vi "20151004 Main_one action input .vi"() -> ()   [LabVIEW 2013]
uses:
  SSNN(super simple neural network)_2.1/Neural Network/Types/Stop Settings.ctl
  SSNN(super simple neural network)_2.1/Neural Network/Types/Error Evaluation.ctl
  <vilib>/MakerHub/LINX/Public/Sensors/Accelerometer/MPU60X0/DeviceAddresses.ctl
  controls/20151109 Action set.ctl
  controls/Pulse limit.ctl
  controls/Sample set.ctl
  SSNN(super simple neural network)_2.1/Neural Network/Types/Teaching Vector.ctl
  SSNN(super simple neural network)_2.1/Neural Network/Types/1D Array.ctl
  SSNN(super simple neural network)_2.1/Neural Network/Types/Neural Network.ctl
  SSNN(super simple neural network)_2.1/Neural Network/Types/2D Array.ctl
  SSNN(super simple neural network)_2.1/Neural Network/Types/Scaling Info.ctl
  SSNN(super simple neural network)_2.1/Neural Network/Super Simple Neural Network.lvlib
  <vilib>/MakerHub/LINX/Public/Sensors/Accelerometer/MPU60X0/MPU60X0.lvlib
panel:
  in  "Pulse limit":T1={"Pulse upper limit"=2400, "Pulse lower limit"=1500, "Fuzzy range"=50.0}
  out "Action chart":i16(graph)
  in  "Initial Pulse Widths (uS)":u16[](array[numeric])=[1100, 900, 2100, 1500, 1500, 600, 1600, 2100, 600, 1400, 700, 600] min=600 max=2400 step=100
  in  "Actions":T2=[-100, -50, -10, 0, 10, 50, 100]
  out "Pitch&Roll":T3(graph)={"Pitch"=1.64306105519083, "Roll"=-26.60639904187085, "Pulse"=1500.0, "Action"=0.0, "Pitch'"=0.0, "Roll'"=0.0, "Pulse'"=0.0}
  in  "Q learning setting":T4={"Pitch +limit"=15.0, "Pitch -limit"=-15.0, "Roll +limit"=5.0, "Roll -limit"=0.0, "Cost_c"=0.01, "Cost_0"=0.0, "Discounting factor"=1.0} {"Cost_0" format="%#_13g"; "Cost_c" format="%#_13g"}
  out "Cycles":i32=599
  in  "Neural network setting":T5={"Add Bias Inputs"=TRUE, "Output Layer Linear"=FALSE, "1st Hidden Layer"=10, "2nd Hidden Layer"=10, "# Inputs"=4, "Output Neurons/Outputs"=1}
  out "Error Trend":dbl[](graph)=[333.88049946998603, 84.67257917593295, 79.55145375361836, 165.88618567000654, 164.395409026523, 66.2860419585734, 89.94237535998712, 89.31153569817062, 48.467858482266436, 75.00403729966206, 75.0129349957244, 53.15644774430287, 49.173023491017965, 48.64104572122034, 47.03615785475572, 56.77040737122186, 56.73707087203033, 50.66515759517278, 46.94108756608759, 47.05005218060951, 49.10730725338338, 50.14010228928986, 49.105932754914605, 47.54849782076006, 46.130158362809, 45.14431666029949, 44.40933619615308, 43.21622556663465, 39.5637978090232, 41.311588761627874, 36.04355325175722, 32.85251820100693, 32.65212220800668, 28.980505575795966, 24.613605659371288, 22.04828944280029, 33.15201456870398, 19.751806387640762, 24.983784772589345, 20.123556544702225, 22.16816710032048, 24.761419168572694, 20.519403969578008, 22.075445422683597, 20.68097799083518, 21.774609704131727, 21.601837537514506, 21.08381595647031, 20.43182890729097, 22.04427690550854, 20.894295129000575, 20.106993070447466, 20.890368283068455, 21.208917859881538, 20.63770876867939, 21.091536913629373, 20.998527289682343, 20.795457971936926, 21.02597611803169, 20.227157731616355, 21.215734162324786, 20.650262532179397, 21.005392179444087, 20.725327488997934, 20.687878356478905, 20.855553191124425, 20.801611756610075, 20.738643649346614, 20.688105294347146, 20.838851997630606, 20.684708818314576, 20.743170247078012, 20.838027711435757, 20.914507377770732, 20.67245494693975, 21.54523281643815, 20.0435987021579, 20.88854916583944, 21.20680684383158, 20.85298901480824, 20.945538137596667, 21.117452737900226, 21.17987166719355, 21.255397820084887, 20.445274173192253, 21.195173705398183, 21.313235473119207, 20.029865394337943, 20.585349566646947, 21.355689354848963, 20.960316068407973, 20.761365861531807, 20.606789221792013, 20.558601442864358, 20.835972008235984, 21.022960041760562, 20.841389775063547, 20.81595335032675, 20.838171160161544, 20.927269052498737, 21.071870765314067, 21.134653122269086, 20.883207609643364, 21.128088298885018, 21.655842540724205, 20.102655683916797, 21.72496471296433, 21.50337264288738, 21.012302171905347, 21.621733979373943, 20.272540939113394, 20.96004746440345, 21.00549114787492, 20.738198000636928, 20.90456052208629, 21.09783104667723, 20.802636011566328, 20.72196563917106, 20.88459613344823, 21.034990278462956, 20.965840529107496, 21.09943451012232, 20.841270113600014, 22.248500578009008, 21.252361413765815, 21.23455803466164, 21.537219762358855, 21.074723451111687, 20.93522564988776, 21.07809401987224, 21.17671611661583, 20.27121832525152, 21.471799828024608, 21.4291887393944, 21.18363971171234, 21.50913451674851, 21.59767834823473, 20.956373553635203, 21.822837431390372, 21.49753461733536, 21.485968082905877, 21.48494245696796, 21.318220512481936, 21.367936043412126, 20.94616048474088, 20.753916097135427, 21.07204391789874, 20.306074221150077, 21.01405471875159, 20.530256721680587, 20.526249130307217, 20.80689321403159, 20.895746298916457, 20.607343338944055, 20.597797231039035, 20.904292837205865, 20.960971747805274, 21.028246046977777, 21.179852554879616, 21.392519030048973, 20.90089495657071, 21.138385592397718, 21.414598513102884, 20.40922445138783, 20.953480526264897, 21.591846597945157, 21.15306743419646, 20.774874247956575, 20.94548496453009, 21.09232518066816, 21.01287861720526, 20.977791815244213, 20.927526645349978, 20.431706129072563, 20.67672182091419, 20.722891703135723, 20.75923618212, 20.357836480756728, 20.389436414993053, 20.10136178717, 20.736898887818544, 20.75206611355616, 20.38895892080945, 20.568167184661817, 20.920533307915083, 20.857038534800424, 20.580083375056084, 20.785103003816396, 20.958122793972255, 20.6544112973137, 20.53535667031042, 20.516752039319098, 20.760368641671185, 20.919917043637327, 20.564170595579625, 20.385856753450483, 20.405711663808006, 20.576591428970247, 20.64437732279147, 20.682686671745024, 50.109218416394455, 48.68659907551151, 24.291876984471525, 23.82831185269545, 23.75818920903926, 22.928862712340567, 21.98058417644527, 20.917149195880697, 20.132785560581155, 20.169437998270386, 20.578950065032494, 21.008224203211334, 20.906061374122352, 20.725896421086105, 20.579350890353826, 20.554285162206753, 20.592781147960377, 20.63897403541673, 20.694443280446805, 20.677897032394593, 20.704340499261313, 20.747705833484325, 20.85133518407087, 20.665980162241137, 20.802009113403784, 20.97590970878443, 20.873861827068318, 20.86882085443502, 21.142178961512435, 20.888114949143322, 20.79039166740166, 20.91726119020472, 20.981407674757513, 21.070293162022054, 20.871359933527465, 21.1696423771655, 20.958911563993276, 21.138818620736476, 21.188745483796453, 21.061489493387555, 21.196260749824575, 21.416474482804347, 21.28216705177759, 21.138216742593812, 21.191299004700852, 21.267383294997007, 21.276223845987765, 21.214794549776222, 21.159289147691318, 21.233647898029737, 21.24171547279363, 21.256142303435578, 21.277336990075746, 21.25844818529064, 21.231920861570494, 21.40242475570374, 21.321251366378597, 21.29612606710706, 21.45791961570138, 21.367477977274458, 21.37268365681034, 21.40341592914168, 21.349075692799452, 21.32582576745405, 21.41901766989573, 21.304601575091404, 21.35466812407349, 21.188179606013094, 21.356286488369584, 21.37457959015183, 21.0993217241719, 21.402894633993718, 21.489947304379722, 21.540715402245105, 21.410518782567383, 21.38046485668289, 21.474846903988393, 21.31898077504355, 21.455523616927625, 21.52465387397073, 21.44061595372178, 21.421504516036897, 21.408915039105366, 21.401206766536543, 21.395649043373695, 21.391883152471102, 21.395588958273162, 21.55712791809154, 21.34443716294099, 21.464640702604573, 21.373825472290232, 21.368394877234685, 21.273400161951354, 21.381769037159792, 21.504057034310623, 21.431109434849343, 21.406356563823177, 23.65540205511229, 22.810992722631568, 20.57923899988198, 20.58319007676082, 20.81263150913389, 21.170869056468376, 21.379224044692158, 21.37629298836194, 21.213295459842634, 21.230438315361745, 21.325758742290823, 21.354394013075165, 21.211063321275766, 21.0843295287686, 21.103745599801687, 21.138072677749115, 21.157544205733323, 21.146932569775494, 21.139536014739676, 21.134917818609246, 21.131171728890486, 21.13010683574455, 21.08863070003151, 21.072473100037904, 21.052648771003255, 21.191602127550013, 21.189717554146938, 21.13037110867332, 21.106376286286423, 21.081745588813632, 21.057196835718134, 20.961595462095396, 21.017616938516692, 20.760256244853846, 20.805420114150202, 20.726709372920546, 20.72566916555688, 20.762960179962377, 20.600915888471803, 20.723000104170623, 21.206529558160877, 20.2743675240325, 20.224319463723184, 20.384460691153343, 20.51660393741115, 20.459834880296683, 20.393339130553915, 20.335910014816854, 20.32231007375009, 20.30070730148315, 20.292780662800347, 20.328729450966357, 20.305267245409468, 20.3252314329303, 20.33282820701112, 20.34285833144068, 20.269442551533906, 20.14519288440736, 20.11158095395371, 20.139926775184698, 20.032978502368678, 19.999520398198612, 19.96351766289139, 20.03809953441751, 20.160870265578325, 20.482927098545208, 20.130926729621876, 20.09725914077078, 20.100238495818097, 20.116583568620168, 19.95914544590437, 19.94071716708422, 19.940300964376128, 19.98599051881476, 20.078609366082595, 20.01307232756259, 19.99978164928349, 20.00302972085362, 19.908651015960583, 19.873822333862336, 19.874973498287304, 19.913149238983777, 20.01952748864808, 20.096695943966417, 20.143768069271964, 20.141383096397952, 20.136831004259925, 20.223149747485653, 20.19905713205555, 20.750847424398764, 20.809736686993276, 20.501775773019872, 20.33442714740368, 20.572605386928966, 20.827668774993178, 20.678658825599985, 20.431138871490077, 20.25901325864845, 20.221797894623343, 20.286842212423792, 20.329531029511124, 20.294444175502328, 20.253428639375635, 20.215813791530792, 20.2050897505637, 20.18308261462991, 20.159070283807253, 20.13228969737459, 20.11173710363827, 20.09101248192082, 20.080421525208493, 20.093890985622465, 20.089194658832106, 20.050043664638643, 20.044272022415278, 20.04952900915421, 20.001427591963555, 19.964392111299475, 19.91597817519235, 19.866619409630758, 19.841378813419944, 19.577993292486816, 19.685341467699523, 19.747359588926592, 19.887379040776874, 19.786655696397272, 19.8072196992904, 19.90985659992834, 19.65888340013998, 19.49619554742913, 19.486913507524626, 19.472186318770902, 19.485409917675618, 19.41815941153705, 19.4054771779139, 19.445348789523074, 19.38062744079263, 19.413440698692874, 19.42521800623132, 19.42256855105356, 19.34476429284491, 19.358493517673445, 19.33704429793075, 19.30716844110046, 19.240965023840126, 19.229904692660355, 19.009769996366423, 19.065703954140808, 19.05148611896066, 19.02280928703337, 18.951406884352046, 18.98511641198081, 18.898378684078615, 18.8668745459602, 18.85121183540422, 18.732357936464517, 18.712393184517445, 18.677874084378182, 18.611120914138617, 18.560663650200375, 18.49595218986611, 18.456735811957824, 18.381795683052637, 18.32128673117479, 18.304023560742543, 18.175967195285637, 18.222868327275993, 18.078582832271884, 18.128511999728396, 18.090366101032338, 17.83461141473602, 17.718425007102372, 17.733743355265418, 17.72123423977747, 17.669166899064358, 17.671123268836503, 17.69635595095116, 17.651703613274016, 17.611210306307086, 17.543912373707315, 17.416376807595938, 17.32014074436058, 17.223286548024703, 17.225275914593773, 17.140880411831326, 16.901251796832625, 16.963859754427617, 17.270605236519025, 17.272528306915063, 17.1765185101457, 17.005045251098373, 16.925584386095224, 16.977890062196234, 17.056402094066613, 17.03291485886513, 16.992870407704256, 16.968543606571032, 16.95047444559997, 16.9402256780742, 16.924399638911176, 16.910498652345275, 16.89368583659985, 16.87873435176578, 16.862582856505863, 16.843313129608877, 16.821385858117925, 16.782582125811373, 16.726810784315255, 16.680272908113288, 16.519954152006775, 16.536373716679687, 16.562482401642868, 16.603640899555582, 16.62179827743067, 16.595817051470714, 16.479323396837113, 16.492128209451277, 16.495199616509865, 16.431366799200475, 16.455173545574457, 16.421571689738734, 16.377118416338263, 16.349049380128818, 16.348552023942062, 16.311626802032794, 16.348413961112485, 16.34040984808371, 16.300522183858632, 16.1844545958049, 16.227120234676107, 16.36823733164011, 16.3724109943891, 16.3022741960022, 16.153436825740613, 16.06170977992999, 16.082417640840237, 16.12085969232318, 16.14497412498674, 16.14890722176546, 16.128907230253166, 16.102116676114218, 16.089009958136856, 16.068110658545915, 16.064743090727617, 16.064792499952702, 16.09715975558004, 16.1390220225545, 16.05560019149494, 16.004515112004757, 16.069098757892437, 16.090484759336753, 16.045355250383608, 16.025231676560402, 16.039623009317324, 15.993588970194892, 15.92515380014044, 15.876480981988767, 15.879984253623178, 15.9102763203441, 15.929495224112808, 15.941134546284838, 15.922569702607708, 15.922305595240468, 15.907815946098271, 15.885004090236592, 15.86343189494666, 15.846698711226622, 15.86328942472962, 15.87514150977072, 15.844903229183537, 15.82953331842107, 15.778735498603012, 15.795926858464746, 15.781056004373271, 15.774130259292837, 15.733095002983731, 15.66395395721543, 15.595468377168253, 15.571055311815932, 15.594800549447452, 15.582911073515067, 15.484237193288545, 15.38985567338683, 15.482044495316837, 15.553501712519163, 15.547188678491967, 15.435123326032336, 15.30063701969776, 15.236856117796512, 15.172174009204562, 15.186367008579237, 15.229150415441268, 15.218947961452974, 15.129199062491393, 15.047379054888552, 15.016631135764975, 14.953760247784125, 14.865431984810913, 14.79087482252337, 14.746318013061174, 14.65656838328891, 14.465197939093837, 14.359935708953522]
  in  "Hard ware config":T7={"Serial Port"="COM10", "Device Address"=enum."0x68", "Servo Channels"=[2, 3, 4, 5, 6, 7, 8, 9, 10, 11, 12, 13]}
  in  "Weights in(Collect con)":path=path "C:/Users/Kuanho/Desktop/Learning Quadruped project/20151116 Learning Quadruped/Data/Weights/20151119"
  in  "Weights in(Best policy)":path=path "C:/Users/Kuanho/Desktop/Learning Quadruped project/20151116 Learning Quadruped/Data/Weights/20151119"
  out "error out":errorcluster
  in  "error in (no error)":errorcluster
  in  "stop":bool=TRUE
  out "Goal Reached":bool
  in  "Termination Settings In":T8={"Max Epocs"=600, "Error Goal"=0.1, "Max Time (s)"=600.0, "Error Evaluation"=enum."Over Teaching Set"}
  in  "Weights out":path=path "C:/Users/Kuanho/Desktop/Learning Quadruped project/20151116 Learning Quadruped/Data/Weights/20151119"
  in  "Transition data in(Learn)":path=path "C:/Users/Kuanho/Desktop/Learning Quadruped project/20151116 Learning Quadruped/Data/Transition data/20151119"
  in  "Weights in(Learn)":path=path "C:/Users/Kuanho/Desktop/Learning Quadruped project/20151116 Learning Quadruped/Data/Weights/20151119"
  in  "Transition data out":path=path "C:/Users/Kuanho/Desktop/Learning Quadruped project/20151116 Learning Quadruped/Data/Transition data/20151119"
  out "Pulse Widths (uS)":u16[](array[numeric])=[1100, 900, 2100, 1500, 1500, 600, 1600, 2100, 600, 1400, 700, 600]
  in  "Cycles":i32=600
  in  "Senario":T10(ring)=enum."Best policy"
  in  "Joint(ch) controled":i32=6
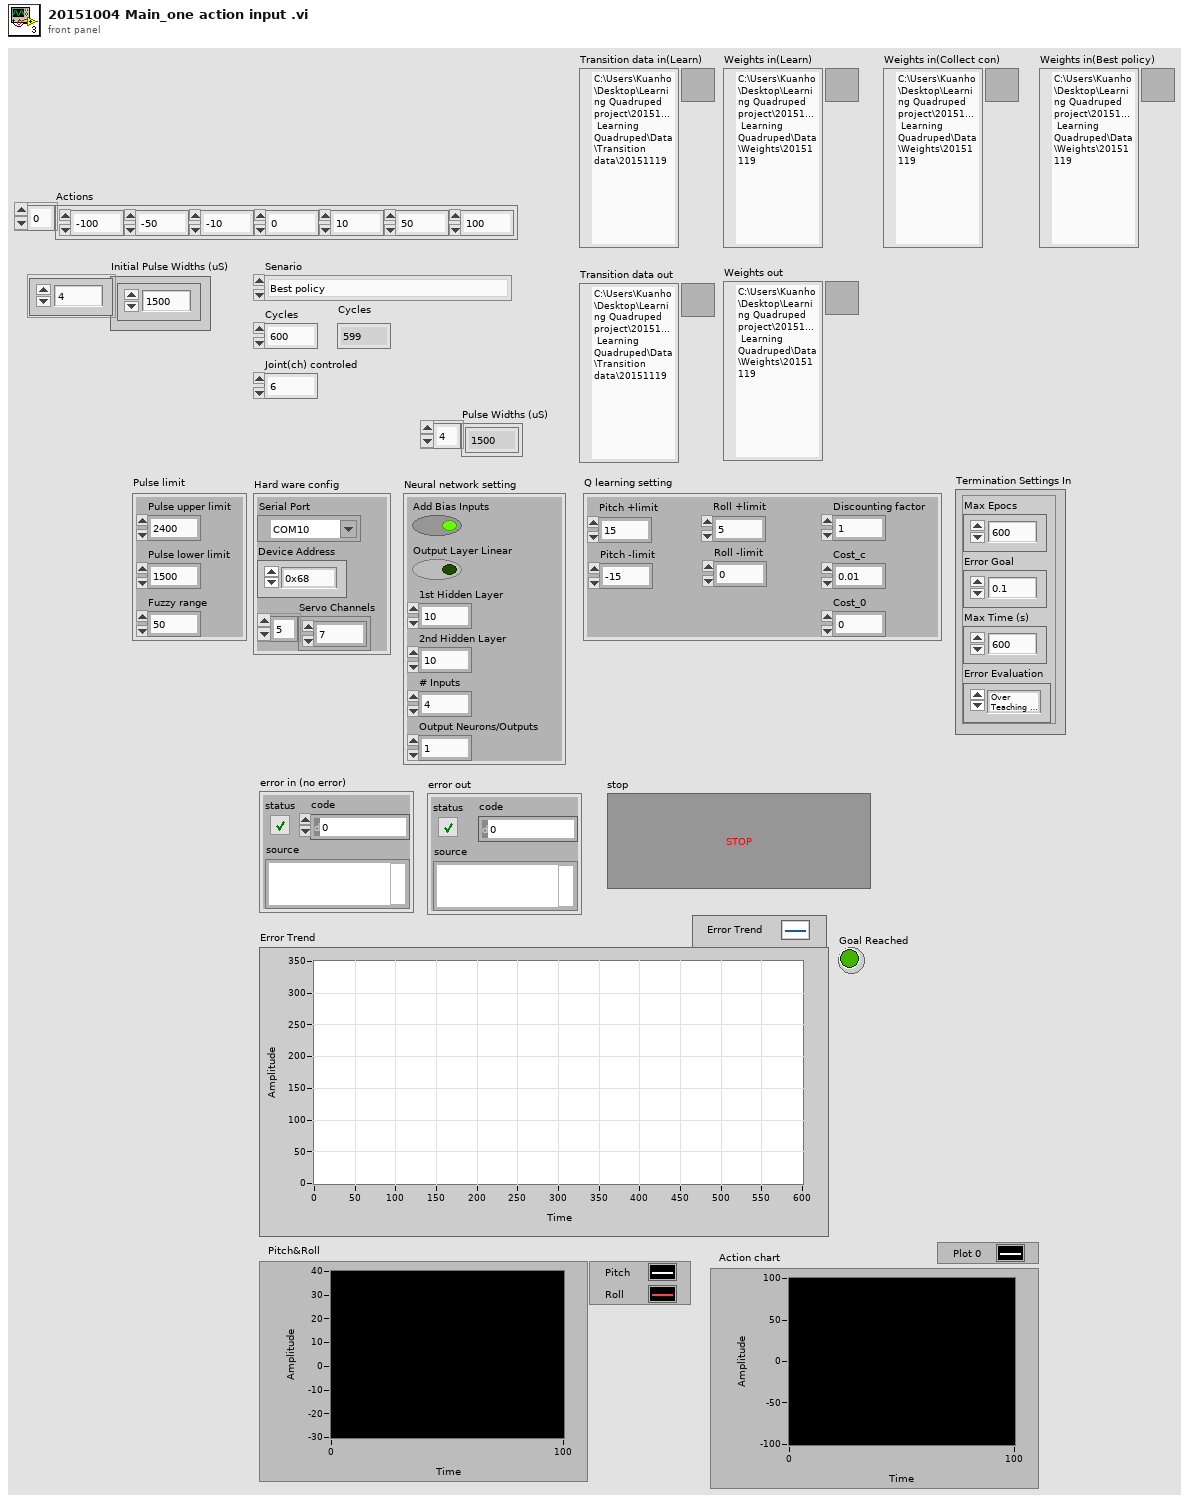
[diagram p1: front panel]
types:
  T1 = typedef "Pulse limit.ctl" = cluster{"Pulse upper limit":i16, "Pulse lower limit":i16, "Fuzzy range":dbl}
  T2 = typedef "20151109 Action set.ctl" = i16[]
  T3 = cluster{"Pitch":dbl, "Roll":dbl, "Pulse":dbl, "Action":dbl, "Pitch'":dbl, "Roll'":dbl, "Pulse'":dbl}
  T4 = cluster{"Pitch +limit":dbl, "Pitch -limit":dbl, "Roll +limit":dbl, "Roll -limit":dbl, "Cost_c":dbl, "Cost_0":dbl, "Discounting factor":dbl}
  T5 = cluster{"Add Bias Inputs":bool, "Output Layer Linear":bool, "1st Hidden Layer":u32, "2nd Hidden Layer":u32, "# Inputs":u32, "Output Neurons/Outputs":u32}
  T6 = typedef "LMH-LINX.lvlib/MPU60X0.lvlib/DeviceAddresses.ctl" = enum16{"0x68", "0x69"}
  T7 = cluster{"Serial Port":refnum<visa-resource-name>, "Device Address":T6, "Servo Channels":u8[]}
  T8 = typedef "Super Simple Neural Network.lvlib/Stop Settings.ctl" = cluster{"Max Epocs":u64, "Error Goal":dbl, "Max Time (s)":dbl, "Error Evaluation":T9}
  T9 = typedef "Super Simple Neural Network.lvlib/Error Evaluation.ctl" = enum16{"Over Both Sets", "Over Validation Set", "Over Teaching Set"}
  T10 = enum16{"Collect data(initial)", "Initialize weights", "Collect data(continue)", "Learn data", "Best policy"}
  T11 = enum16{"Initialize", "Read acc & gyro", "Write servos", "Stop"}
  T12 = typedef "Sample set.ctl" = cluster{"Pitch":dbl, "Roll":dbl, "Pulse":dbl, "Action":dbl, "Pitch'":dbl, "Roll'":dbl, "Pulse'":dbl}
  T13 = typedef "Super Simple Neural Network.lvlib/1D Array.ctl" = cluster{"1D Array":dbl[]}
  T14 = typedef "Super Simple Neural Network.lvlib/Teaching Vector.ctl" = cluster{"Inputs":T13, "Expected Outputs":T13}
  T15 = typedef "Super Simple Neural Network.lvlib/Neural Network.ctl" = cluster{"Weigths":T16[], "Last Layer Linear":bool, "Add Bias Inputs":bool, "# Inputs":u32, "# Output Neurons/Outputs":u32, "Inputs Scaling":T17, "Outputs Scaling":T17}
  T16 = typedef "Super Simple Neural Network.lvlib/2D Array.ctl" = cluster{"2D Array":dbl[][]}
  T17 = typedef "Super Simple Neural Network.lvlib/Scaling Info.ctl" = cluster{"X Scaling Vector":dbl[], "Y Scaling Vector":dbl[]}
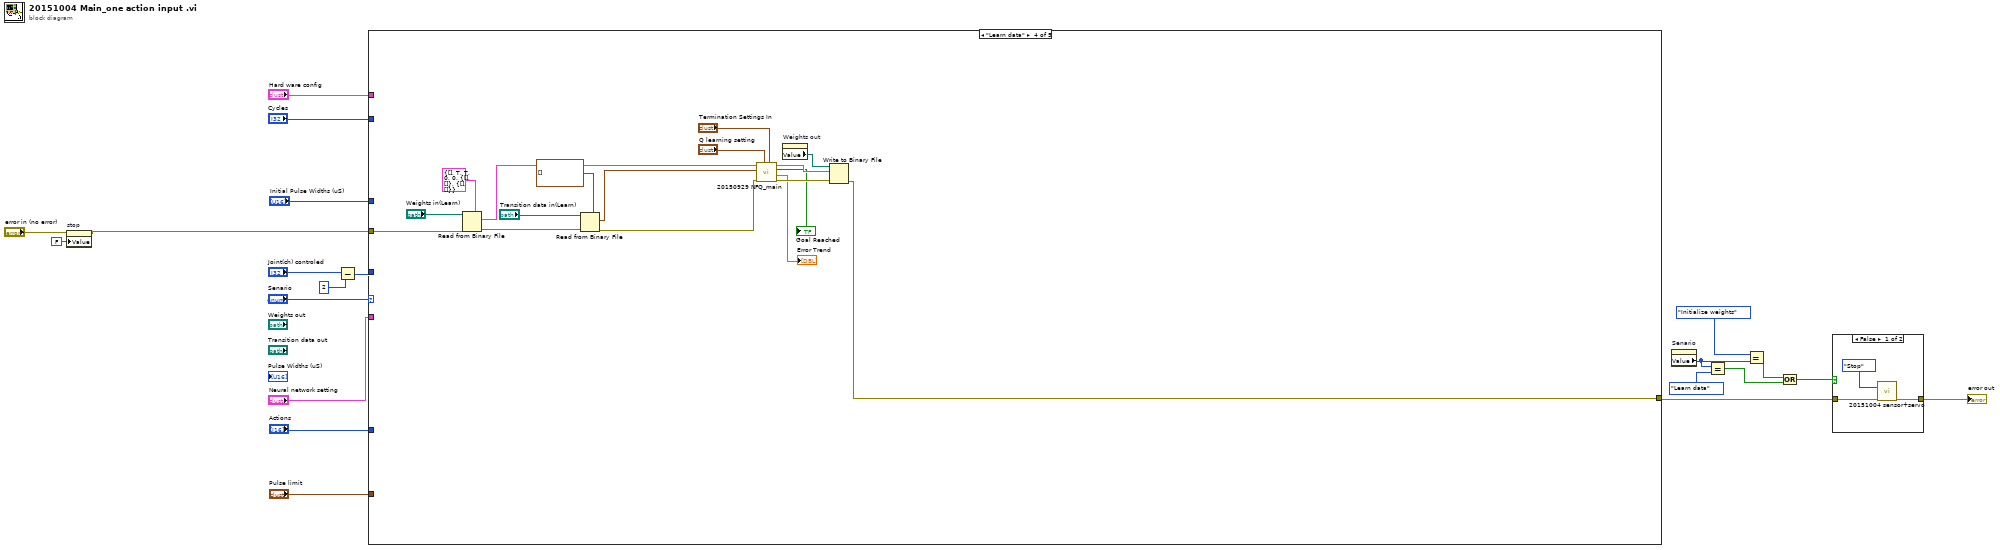
[diagram p0: block diagram]
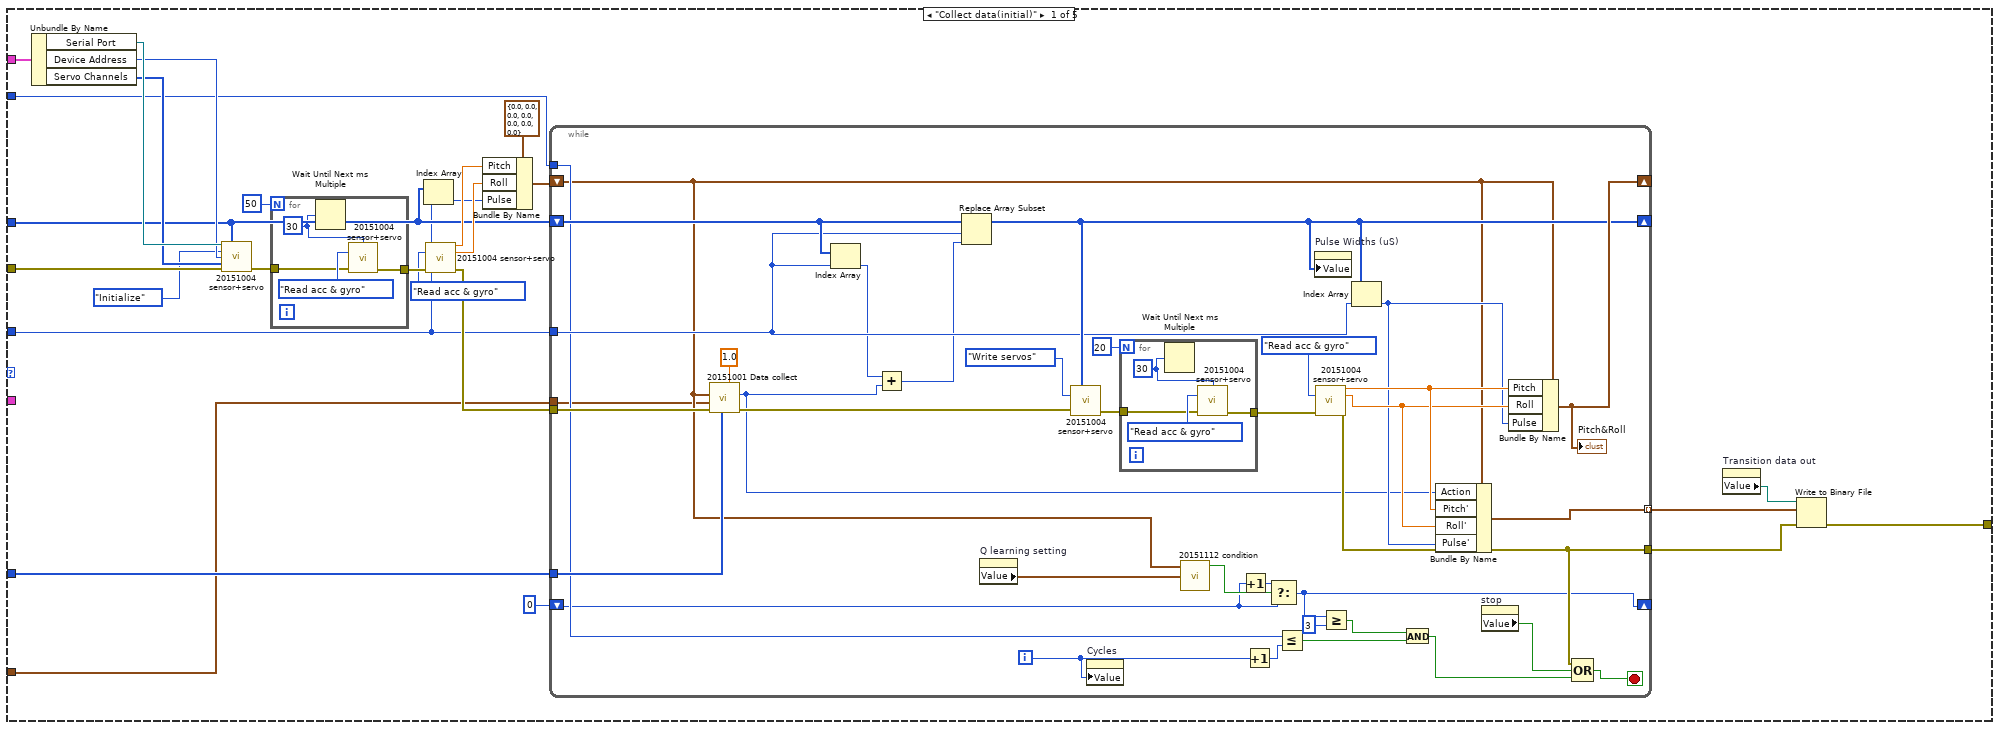
[diagram p3: hidden frame]
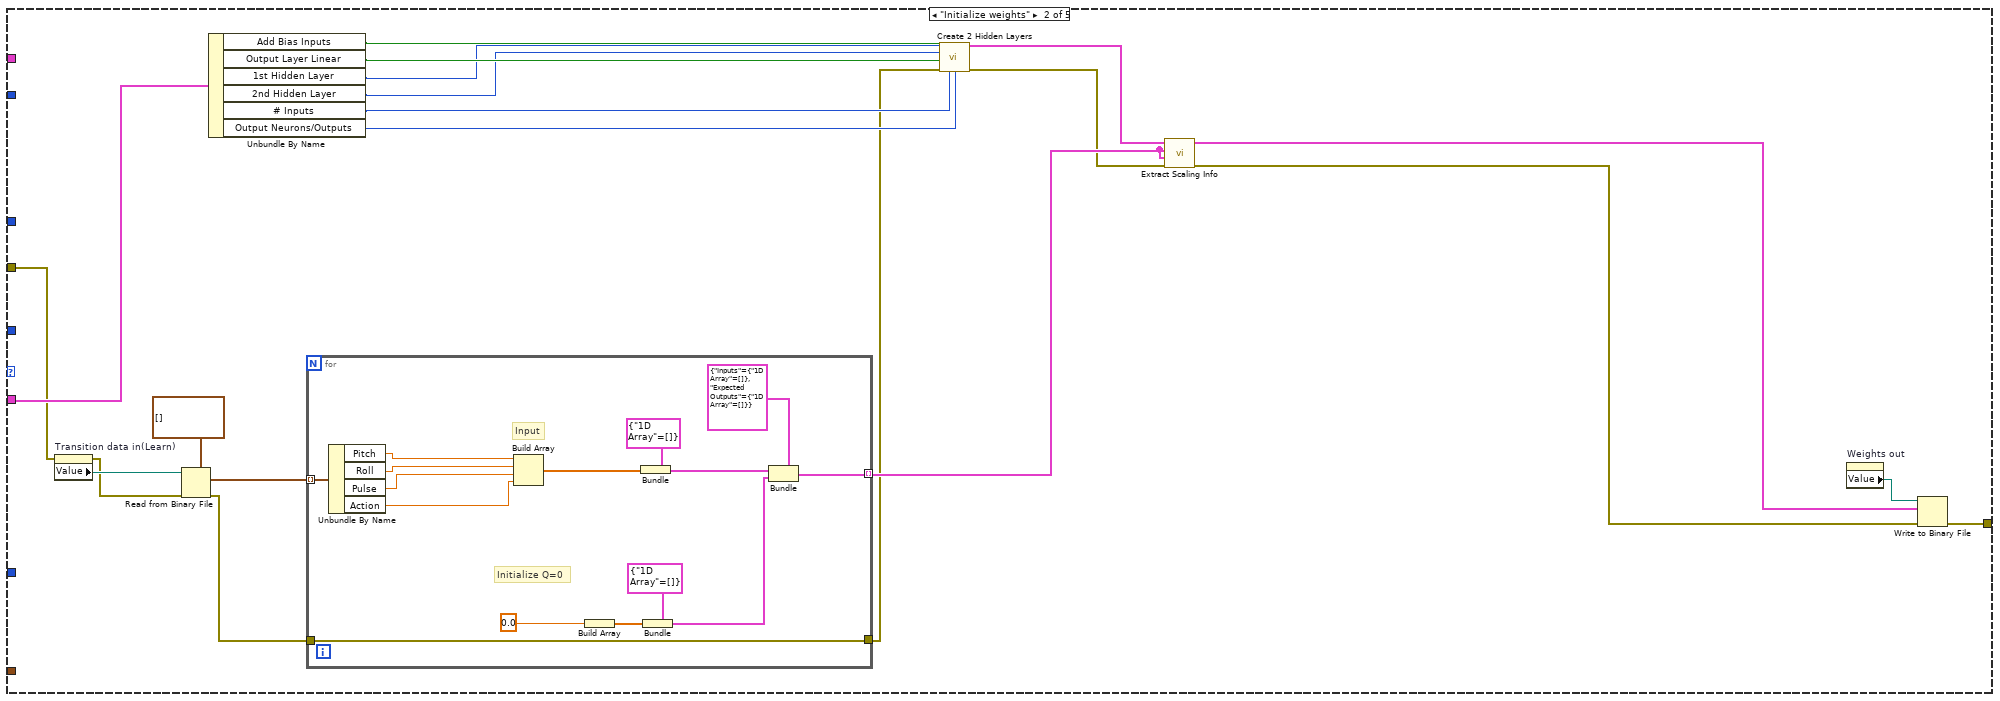
[diagram p4: hidden frame]
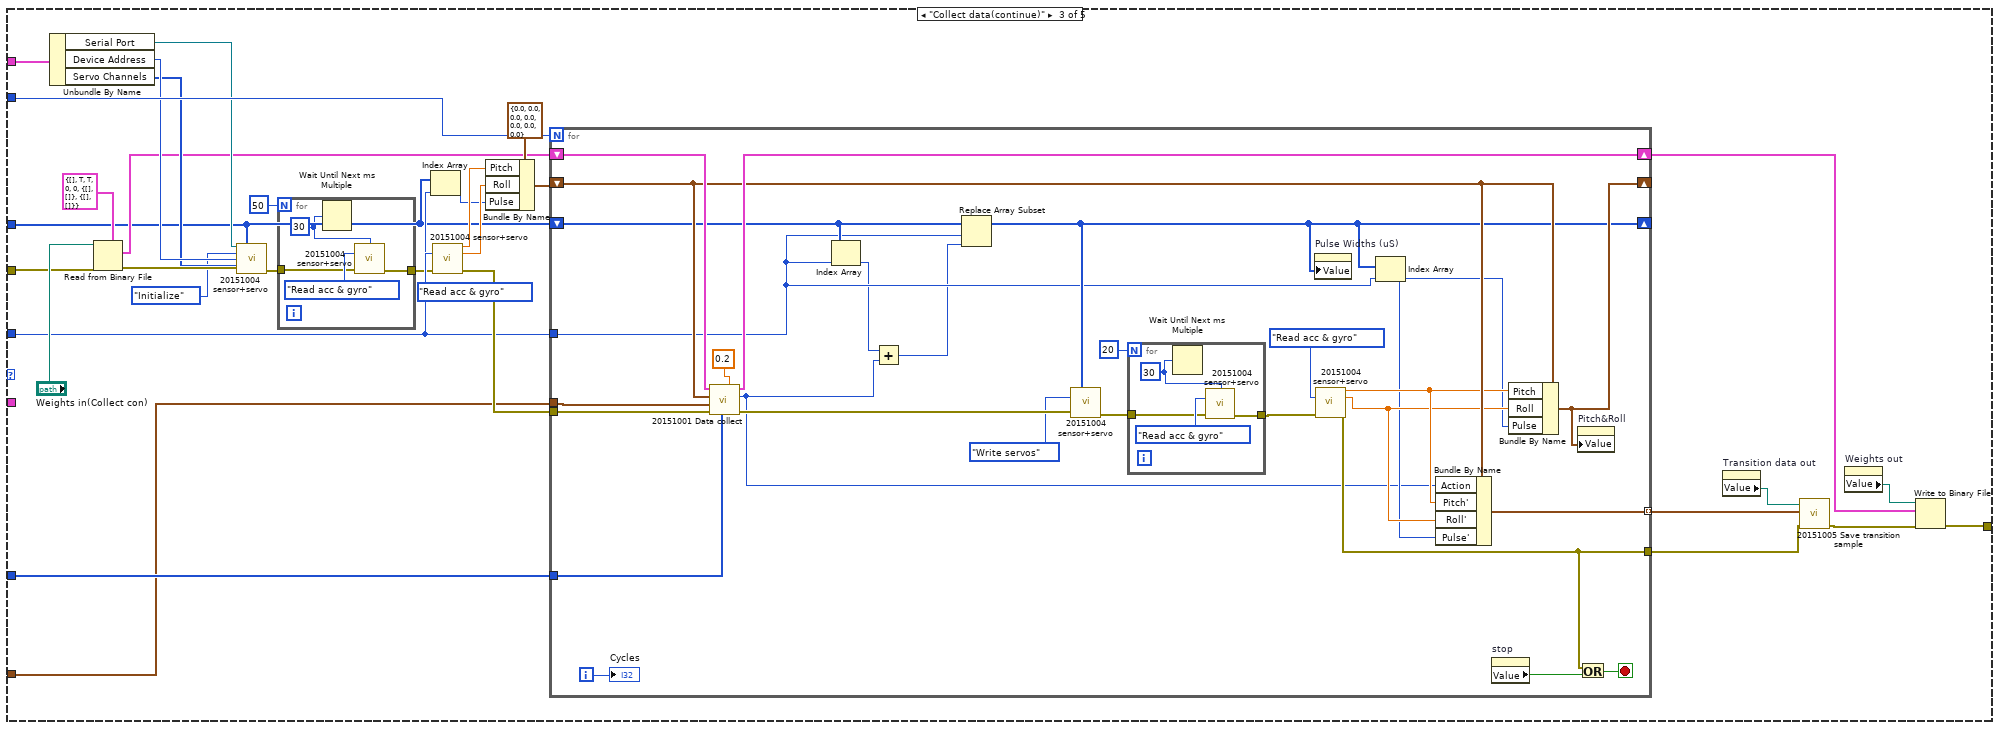
[diagram p5: hidden frame]
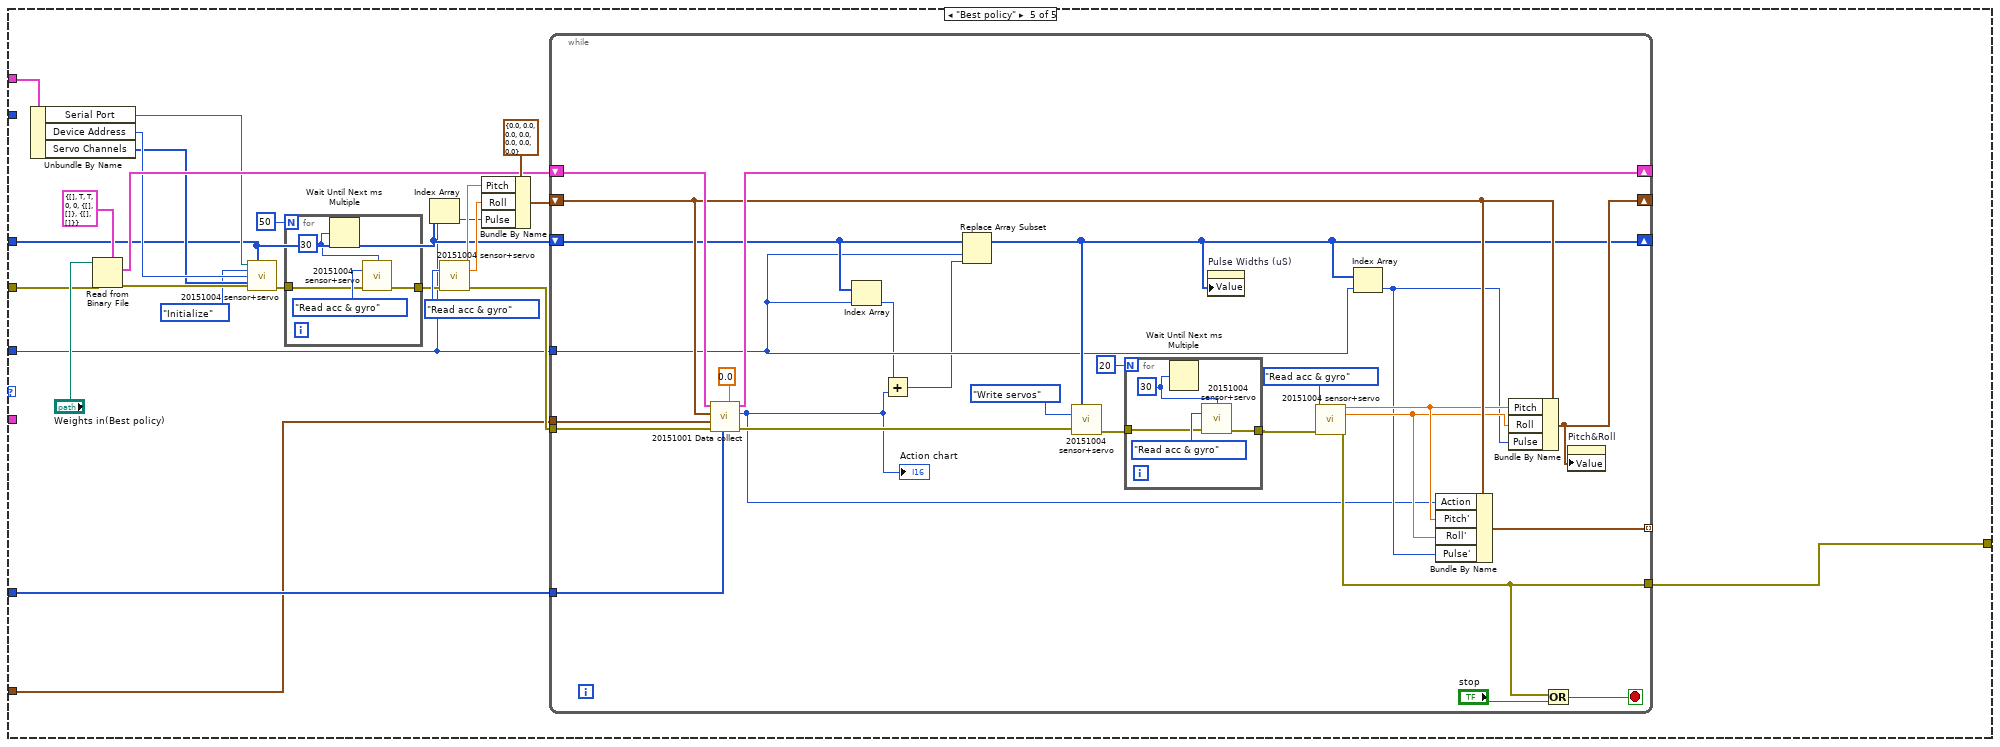
[diagram p6: hidden frame]
diagram:
  n1 = property on="stop" class="Bool (strict)"(error in="error in (no error)", "Value"=FALSE ("stop")) -> (error out=w17:errorcluster)  [unwired: 1 in, 1 out]
  n2 = Subtract(x="Joint(ch) controled", y=2) -> (x-y=w12:i32)
  n3 = case shown="\"Learn data\"" "Senario" {
    tunnel: "Initial Pulse Widths (uS)" -> [w28 _ w130 _ w216]
    tunnel: "Cycles" -> [w24 _ w158 _ _]
    tunnel: w12 -> [w26 _ w131 _ w215]
    tunnel: w17 -> [w41 w102 w155 w202 w233]
    tunnel: [w25 w112 w148 w208 w236] -> w14
    tunnel: "Hard ware config" -> [w45 _ w153 _ w227]
    tunnel: "Neural network setting" -> [_ w106 _ _ _]
    tunnel: "Actions" -> [w35 _ w140 _ w225]
    tunnel: "Pulse limit" -> [w22 _ w129 _ w214]
    frame "Collect data(initial)" {
      n4 = Unbundle By Name(w45) -> ("Serial Port"=w44:refnum<visa-resource-name>, "Device Address"=w43:T6, "Servo Channels"=w42:u8[])
      n5 = call "20151004 sensor+servo.vi"("Serial Port"=w44, "Pulse Widths (uS)"=w28, "Action(hardware)"=T11."Initialize", "Device Address"=w43, "Servo Channels"=w42, "error in (no error)"=w41) -> ("Error Out"=w36:errorcluster)  [unwired: 6 in, 3 out]
      n6 = for {
        N: 50 -> [_]
        tunnel: w36 -> [w91]
        tunnel: [w90] -> w33
        w89 = u32 30 ("millisecond multiple")
        n7 = Wait Until Next ms Multiple(millisecond multiple=w89) -> ()  [unwired: 1 out]
        n8 = call "20151004 sensor+servo.vi"("Loop time"=w89, "Action(hardware)"=T11."Read acc & gyro", "error in (no error)"=w91) -> ("Error Out"=w90:errorcluster)  [unwired: 9 in, 3 out]
      }
      n9 = Index Array(array=w28, index=w26) -> (element=w27:u16)
      n10 = call "20151004 sensor+servo.vi"("Action(hardware)"=T11."Read acc & gyro", "error in (no error)"=w33) -> ("pitch"=w30:dbl, "roll"=w29:dbl, "Error Out"=w32:errorcluster)  [unwired: 10 in, 1 out]
      n11 = Bundle By Name(cluster=T12 {"Pitch"=0.0, "Roll"=0.0, "Pulse"=0.0, "Action"=0.0, "Pitch'"=0.0, "Roll'"=0.0, "Pulse'"=0.0} ("Sample set"), "Pitch"=w30, "Roll"=w29, "Pulse"=w27) -> (w46:T12)
      n12 = while {
        tunnel: w32 -> [w84]
        shift-right: [w69] -> _
        shift-left: w28 -> [w67]
        tunnel: w26 -> [w66]
        shift-right: [w70] -> _
        shift-left: w46 -> [w60]
        tunnel: [w82] -> w38 mode=indexing
        tunnel: [w78] -> w37
        tunnel: w35 -> [w64]
        tunnel: w24 -> [w63]
        shift-right: [w55] -> _
        shift-left: 0 -> [w57]
        tunnel: w22 -> [w48]
        i -> [w51]
        stop <- w80 stop-if-true
        n13 = call "20151001 Data collect.vi"("Epilson(Explore probability )"=1.0, "Actions"=w64, "Error In"=w84, "Pulse limit"=w48, "Sample set"=w60) -> ("Error Out"=w83:errorcluster, "Action"=w50:i16)  [unwired: 4 in, 1 out]
        n14 = Index Array(array=w67, index=w66) -> (element=w65:u16)
        n15 = Add(x=w65, y=w50) -> (x+y=w49:u16)
        n16 = Replace Array Subset(array=w67, new element=w49, index=w66) -> (w69:u16[])
        n17 = property on="Q learning setting" class="Clust (strict)"() -> ("Value"=w61:T4)  [unwired: 2 in, 2 out]
        n18 = call "20151004 sensor+servo.vi"("Pulse Widths (uS)"=w69, "Action(hardware)"=T11."Write servos", "error in (no error)"=w83) -> ("Error Out"=w72:errorcluster)  [unwired: 9 in, 3 out]
        n19 = property on="Cycles" class="DigNum (strict)"("Value"=w51) -> ()  [unwired: 2 in, 2 out]
        n20 = for {
          N: 20 -> [_]
          tunnel: w72 -> [w87]
          tunnel: [w86] -> w71
          w85 = u32 30 ("millisecond multiple")
          n21 = Wait Until Next ms Multiple(millisecond multiple=w85) -> ()  [unwired: 1 out]
          n22 = call "20151004 sensor+servo.vi"("Loop time"=w85, "Action(hardware)"=T11."Read acc & gyro", "error in (no error)"=w87) -> ("Error Out"=w86:errorcluster)  [unwired: 9 in, 3 out]
        }
        n23 = call "20151112 condition.vi"("Condition"=w61, "State"=w60) -> ("result"=w59:bool)  [unwired: 3 in]
        n24 = Increment(x=w57) -> (x+1=w58:i32)
        n25 = Increment(x=w51) -> (x+1=w62:i32)
        n26 = Select(t=w58, s=w59, f=w57) -> (s? t:f=w55:i32)
        n27 = Less Or Equal?(x=w63, y=w62) -> (x <= y?=w56:bool)
        n28 = property on="Pulse Widths (uS)" class="Arr (strict)"("Value"=w69) -> ()  [unwired: 2 in, 2 out]
        n29 = call "20151004 sensor+servo.vi"("Action(hardware)"=T11."Read acc & gyro", "error in (no error)"=w71) -> ("pitch"=w75:dbl, "roll"=w74:dbl, "Error Out"=w78:errorcluster)  [unwired: 10 in, 1 out]
        n30 = Greater Or Equal?(x=w55, y=3) -> (x >= y?=w53:bool)
        n31 = Index Array(array=w69, index=w66) -> (element=w68:u16)
        n32 = And(x=w53, y=w56) -> (x .and. y?=w52:bool)
        n33 = Bundle By Name(cluster=w60, "Action"=w50, "Pitch'"=w75, "Roll'"=w74, "Pulse'"=w68) -> (w82:T12)
        n34 = property on="stop" class="Bool (strict)"() -> ("Value"=w79:bool)  [unwired: 2 in, 2 out]
        n35 = Bundle By Name(cluster=w60, "Pitch"=w75, "Roll"=w74, "Pulse"=w68) -> (w70:T12)
        "Pitch&Roll" <- w70
        n36 = Compound Arithmetic op=OR(w78, w79, w52) -> (w80:bool)
      }
      n37 = property on="Transition data out" class="Path"() -> ("Value"=w39:path)  [unwired: 2 in, 2 out]
      n38 = Write to Binary File(file (use dialog)=w39, data=w38, error in=w37) -> (error out=w25:errorcluster)  [unwired: 3 in, 2 out]
    }
    frame "Initialize weights" {
      n39 = property on="Transition data in(Learn)" class="Path"(error in=w102) -> (error out=w101:errorcluster, "Value"=w103:path)  [unwired: 1 in, 1 out]
      n40 = Read from Binary File(5:T12[] [] ("Data"), 8:w101, 11:w103) -> (0:w100:errorcluster, 2:w99:T12[])  [unwired: 3 in, 2 out]
      n41 = Unbundle By Name(w106) -> ("Add Bias Inputs"=w111:bool, "Output Layer Linear"=w110:bool, "1st Hidden Layer"=w109:u32, "2nd Hidden Layer"=w108:u32, "# Inputs"=w107:u32, "Output Neurons/Outputs"=w105:u32)
      n42 = for {
        tunnel: w99 -> [w122] mode=indexing
        tunnel: w100 -> [w121]
        tunnel: [w121] -> w97
        tunnel: [w116] -> w98 mode=indexing
        # "Initialize Q=0"
        # "Input"
        n43 = Unbundle By Name(w122) -> ("Pitch"=w120:dbl, "Roll"=w119:dbl, "Pulse"=w118:dbl, "Action"=w117:dbl)
        n44 = Build Array(w120, w119, w118, w117) -> (w125:dbl[])
        n45 = Build Array(0.0) -> (w114:dbl[])
        n46 = Bundle(cluster=T13 {"1D Array"=[]} ("Inputs"), "1D Array"=w125) -> (w126:T13)
        n47 = Bundle(cluster=T13 {"1D Array"=[]} ("Expected Outputs"), "1D Array"=w114) -> (w124:T13)
        n48 = Bundle(cluster=T14 {"Inputs"={"1D Array"=[]}, "Expected Outputs"={"1D Array"=[]}}, "Inputs"=w126, "Expected Outputs"=w124) -> (w116:T14)
      }
      n49 = call "Create 2 Hidden Layers.vi"("1st Hidden Layer Neurons"=w109, "Output Layer Linear"=w110, "Add Bias Inputs"=w111, "2nd Hidden Layer Neurons"=w108, "Error In"=w97, "# Inputs"=w107, "Output Neurons/Outputs"=w105) -> ("Neural Network"=w94:T15, "Error Out"=w96:errorcluster)  [unwired: 7 in]
      n50 = call "Extract Scaling Info.vi"("Error In"=w96, "Validation Set In"=w98, "Teaching Set In"=w98, "Neural Network In"=w94) -> ("Error Out"=w95:errorcluster, "Neural Network Out"=w93:T15)  [unwired: 4 in, 2 out]
      n51 = property on="Weights out" class="Path"() -> ("Value"=w113:path)  [unwired: 2 in, 2 out]
      n52 = Write to Binary File(file (use dialog)=w113, data=w93, error in=w95) -> (error out=w112:errorcluster)  [unwired: 3 in, 2 out]
    }
    frame "Collect data(continue)" {
      n53 = Unbundle By Name(w153) -> ("Serial Port"=w152:refnum<visa-resource-name>, "Device Address"=w151:T6, "Servo Channels"=w150:u8[])
      n54 = Read from Binary File(5:T15 {"Weigths"=[], "Last Layer Linear"=TRUE, "Add Bias Inputs"=TRUE, "# Inputs"=0, "# Output Neurons/Outputs"=0, "Inputs Scaling"={"X Scaling Vector"=[], "Y Scaling Vector"=[]}, "Outputs Scaling"={"X Scaling Vector"=[], "Y Scaling Vector"=[]}} ("Neural Network out"), 8:w155, 11:"Weights in(Collect con)") -> (0:w154:errorcluster, 2:w146:T15)  [unwired: 3 in, 2 out]
      n55 = call "20151004 sensor+servo.vi"("Serial Port"=w152, "Pulse Widths (uS)"=w130, "Action(hardware)"=T11."Initialize", "Device Address"=w151, "Servo Channels"=w150, "error in (no error)"=w154) -> ("Error Out"=w137:errorcluster)  [unwired: 6 in, 3 out]
      n56 = for {
        N: 50 -> [_]
        tunnel: w137 -> [w163]
        tunnel: [w162] -> w136
        w161 = u32 30 ("millisecond multiple")
        n57 = Wait Until Next ms Multiple(millisecond multiple=w161) -> ()  [unwired: 1 out]
        n58 = call "20151004 sensor+servo.vi"("Loop time"=w161, "Action(hardware)"=T11."Read acc & gyro", "error in (no error)"=w163) -> ("Error Out"=w162:errorcluster)  [unwired: 9 in, 3 out]
      }
      n59 = Index Array(array=w130, index=w131) -> (element=w132:u16)
      n60 = call "20151004 sensor+servo.vi"("Action(hardware)"=T11."Read acc & gyro", "error in (no error)"=w136) -> ("pitch"=w134:dbl, "roll"=w133:dbl, "Error Out"=w135:errorcluster)  [unwired: 10 in, 1 out]
      n61 = Bundle By Name(cluster=T12 {"Pitch"=0.0, "Roll"=0.0, "Pulse"=0.0, "Action"=0.0, "Pitch'"=0.0, "Roll'"=0.0, "Pulse'"=0.0} ("Sample set"), "Pitch"=w134, "Roll"=w133, "Pulse"=w132) -> (w159:T12)
      n62 = for {
        N: w158 -> [_]
        tunnel: w135 -> [w192]
        shift-right: [w172] -> _
        shift-left: w130 -> [w170]
        tunnel: w131 -> [w169]
        shift-right: [w173] -> _
        shift-left: w159 -> [w187]
        shift-right: [w189] -> w147
        shift-left: w146 -> [w190]
        tunnel: [w188] -> w142 mode=indexing
        tunnel: [w183] -> w143
        tunnel: w140 -> [w179]
        tunnel: w129 -> [w166]
        i -> [w180]
        stop <- w185 stop-if-true
        n63 = call "20151001 Data collect.vi"("Epilson(Explore probability )"=0.2, "Actions"=w179, "Error In"=w192, "Pulse limit"=w166, "Sample set"=w187, "Neural Network in"=w190) -> ("Error Out"=w191:errorcluster, "Action"=w167:i16, "Neural Network out"=w189:T15)  [unwired: 3 in]
        n64 = Index Array(array=w170, index=w169) -> (element=w168:u16)
        n65 = Add(x=w168, y=w167) -> (x+y=w165:u16)
        n66 = Replace Array Subset(array=w170, new element=w165, index=w169) -> (w172:u16[])
        n67 = call "20151004 sensor+servo.vi"("Pulse Widths (uS)"=w172, "Action(hardware)"=T11."Write servos", "error in (no error)"=w191) -> ("Error Out"=w175:errorcluster)  [unwired: 9 in, 3 out]
        n68 = for {
          N: 20 -> [_]
          tunnel: w175 -> [w195]
          tunnel: [w194] -> w174
          w193 = u32 30 ("millisecond multiple")
          n69 = Wait Until Next ms Multiple(millisecond multiple=w193) -> ()  [unwired: 1 out]
          n70 = call "20151004 sensor+servo.vi"("Loop time"=w193, "Action(hardware)"=T11."Read acc & gyro", "error in (no error)"=w195) -> ("Error Out"=w194:errorcluster)  [unwired: 9 in, 3 out]
        }
        n71 = property on="Pulse Widths (uS)" class="Arr (strict)"("Value"=w172) -> ()  [unwired: 2 in, 2 out]
        n72 = call "20151004 sensor+servo.vi"("Action(hardware)"=T11."Read acc & gyro", "error in (no error)"=w174) -> ("pitch"=w178:dbl, "roll"=w177:dbl, "Error Out"=w183:errorcluster)  [unwired: 10 in, 1 out]
        n73 = Index Array(array=w172, index=w169) -> (element=w171:u16)
        n74 = Bundle By Name(cluster=w187, "Action"=w167, "Pitch'"=w178, "Roll'"=w177, "Pulse'"=w171) -> (w188:T12)
        n75 = property on="stop" class="Bool (strict)"() -> ("Value"=w184:bool)  [unwired: 2 in, 2 out]
        n76 = Bundle By Name(cluster=w187, "Pitch"=w178, "Roll"=w177, "Pulse"=w171) -> (w173:T12)
        n77 = property on="Pitch&Roll" class="WFChart (strict)"("Value"=w173) -> ()  [unwired: 2 in, 2 out]
        n78 = Or(x=w183, y=w184) -> (x .or. y?=w185:bool)
        "Cycles" <- w180
      }
      n79 = property on="Transition data out" class="Path"() -> ("Value"=w141:path)  [unwired: 2 in, 2 out]
      n80 = call "20151005 Save transition sample.vi"("error in"=w143, "Data"=w142, "Collect data save pos"=w141) -> ("error out"=w144:errorcluster)  [unwired: 8 in]
      n81 = property on="Weights out" class="Path"() -> ("Value"=w149:path)  [unwired: 2 in, 2 out]
      n82 = Write to Binary File(file (use dialog)=w149, data=w147, error in=w144) -> (error out=w148:errorcluster)  [unwired: 3 in, 2 out]
    }
    frame "Learn data" {
      n83 = Read from Binary File(5:T15 {"Weigths"=[], "Last Layer Linear"=TRUE, "Add Bias Inputs"=TRUE, "# Inputs"=0, "# Output Neurons/Outputs"=0, "Inputs Scaling"={"X Scaling Vector"=[], "Y Scaling Vector"=[]}, "Outputs Scaling"={"X Scaling Vector"=[], "Y Scaling Vector"=[]}} ("Neural Network out"), 8:w202, 11:"Weights in(Learn)") -> (0:w206:errorcluster, 2:w199:T15)  [unwired: 3 in, 2 out]
      n84 = Read from Binary File(5:T12[] [] ("Data"), 8:w206, 11:"Transition data in(Learn)") -> (0:w201:errorcluster, 2:w200:T12[])  [unwired: 3 in, 2 out]
      n85 = call "20150929 NFQ_main.vi"("Termination Settings In"="Termination Settings In", "Q learning setting"="Q learning setting", "Error In"=w201, "Sample set array"=w200, "Neural Network In"=w199) -> ("Error Out"=w213:errorcluster, "Error Trend"=→"Error Trend":dbl[], "Goal Reached"=→"Goal Reached":bool, "Neural Network Out(Q)"=w211:T15)  [unwired: 3 in]
      n86 = property on="Weights out" class="Path"() -> ("Value"=w212:path)  [unwired: 2 in, 2 out]
      n87 = Write to Binary File(file (use dialog)=w212, data=w211, error in=w213) -> (error out=w208:errorcluster)  [unwired: 3 in, 2 out]
    }
    frame "Best policy" {
      n88 = Unbundle By Name(w227) -> ("Serial Port"=w230:refnum<visa-resource-name>, "Device Address"=w229:T6, "Servo Channels"=w228:u8[])
      n89 = Read from Binary File(5:T15 {"Weigths"=[], "Last Layer Linear"=TRUE, "Add Bias Inputs"=TRUE, "# Inputs"=0, "# Output Neurons/Outputs"=0, "Inputs Scaling"={"X Scaling Vector"=[], "Y Scaling Vector"=[]}, "Outputs Scaling"={"X Scaling Vector"=[], "Y Scaling Vector"=[]}} ("Neural Network out"), 8:w233, 11:"Weights in(Best policy)") -> (0:w232:errorcluster, 2:w231:T15)  [unwired: 3 in, 2 out]
      n90 = call "20151004 sensor+servo.vi"("Serial Port"=w230, "Pulse Widths (uS)"=w216, "Action(hardware)"=T11."Initialize", "Device Address"=w229, "Servo Channels"=w228, "error in (no error)"=w232) -> ("Error Out"=w222:errorcluster)  [unwired: 6 in, 3 out]
      n91 = for {
        N: 50 -> [_]
        tunnel: w222 -> [w241]
        tunnel: [w240] -> w221
        w239 = u32 30 ("millisecond multiple")
        n92 = Wait Until Next ms Multiple(millisecond multiple=w239) -> ()  [unwired: 1 out]
        n93 = call "20151004 sensor+servo.vi"("Loop time"=w239, "Action(hardware)"=T11."Read acc & gyro", "error in (no error)"=w241) -> ("Error Out"=w240:errorcluster)  [unwired: 9 in, 3 out]
      }
      n94 = Index Array(array=w216, index=w215) -> (element=w217:u16)
      n95 = call "20151004 sensor+servo.vi"("Action(hardware)"=T11."Read acc & gyro", "error in (no error)"=w221) -> ("pitch"=w219:dbl, "roll"=w218:dbl, "Error Out"=w220:errorcluster)  [unwired: 10 in, 1 out]
      n96 = Bundle By Name(cluster=T12 {"Pitch"=0.0, "Roll"=0.0, "Pulse"=0.0, "Action"=0.0, "Pitch'"=0.0, "Roll'"=0.0, "Pulse'"=0.0} ("Sample set"), "Pitch"=w219, "Roll"=w218, "Pulse"=w217) -> (w237:T12)
      n97 = while {
        shift-right: [w250] -> _
        shift-left: w216 -> [w248]
        tunnel: w215 -> [w247]
        shift-right: [w251] -> _
        shift-left: w237 -> [w265]
        shift-right: [w267] -> _
        shift-left: w231 -> [w268]
        tunnel: [w266] -> _ mode=indexing
        tunnel: [w263] -> w236
        tunnel: w220 -> [w258]
        tunnel: w225 -> [w257]
        tunnel: w214 -> [w243]
        stop <- w261 stop-if-true
        n98 = call "20151001 Data collect.vi"("Epilson(Explore probability )"=0.0, "Actions"=w257, "Error In"=w258, "Pulse limit"=w243, "Sample set"=w265, "Neural Network in"=w268) -> ("Error Out"=w269:errorcluster, "Action"=w245:i16, "Neural Network out"=w267:T15)  [unwired: 3 in]
        "Action chart" <- w245
        n99 = Index Array(array=w248, index=w247) -> (element=w246:u16)
        n100 = Add(x=w246, y=w245) -> (x+y=w244:u16)
        n101 = Replace Array Subset(array=w248, new element=w244, index=w247) -> (w250:u16[])
        n102 = call "20151004 sensor+servo.vi"("Pulse Widths (uS)"=w250, "Action(hardware)"=T11."Write servos", "error in (no error)"=w269) -> ("Error Out"=w253:errorcluster)  [unwired: 9 in, 3 out]
        n103 = for {
          N: 20 -> [_]
          tunnel: w253 -> [w272]
          tunnel: [w271] -> w252
          w270 = u32 30 ("millisecond multiple")
          n104 = Wait Until Next ms Multiple(millisecond multiple=w270) -> ()  [unwired: 1 out]
          n105 = call "20151004 sensor+servo.vi"("Loop time"=w270, "Action(hardware)"=T11."Read acc & gyro", "error in (no error)"=w272) -> ("Error Out"=w271:errorcluster)  [unwired: 9 in, 3 out]
        }
        n106 = property on="Pulse Widths (uS)" class="Arr (strict)"("Value"=w250) -> ()  [unwired: 2 in, 2 out]
        n107 = call "20151004 sensor+servo.vi"("Action(hardware)"=T11."Read acc & gyro", "error in (no error)"=w252) -> ("pitch"=w256:dbl, "roll"=w255:dbl, "Error Out"=w263:errorcluster)  [unwired: 10 in, 1 out]
        n108 = Index Array(array=w250, index=w247) -> (element=w249:u16)
        n109 = Bundle By Name(cluster=w265, "Action"=w245, "Pitch'"=w256, "Roll'"=w255, "Pulse'"=w249) -> (w266:T12)
        n110 = Bundle By Name(cluster=w265, "Pitch"=w256, "Roll"=w255, "Pulse"=w249) -> (w251:T12)
        n111 = Or(x=w263, y="stop") -> (x .or. y?=w261:bool)
        n112 = property on="Pitch&Roll" class="WFChart (strict)"("Value"=w251) -> ()  [unwired: 2 in, 2 out]
      }
    }
  }
  n113 = property on="Senario" class="Enum (strict)"() -> ("Value"=w5:T10)  [unwired: 2 in, 2 out]
  n114 = Equal?(x=w5, y=T10."Learn data" ("Senario")) -> (x = y?=w3:bool)
  n115 = Equal?(x=T10."Initialize weights" ("Senario"), y=w5) -> (x = y?=w4:bool)
  n116 = Or(x=w4, y=w3) -> (x .or. y?=w2:bool)
  n117 = case shown="False" w2 {
    tunnel: [w276 w277] -> w15
    tunnel: w14 -> [w275 w277]
    frame False {
      n118 = call "20151004 sensor+servo.vi"("Action(hardware)"=T11."Stop", "error in (no error)"=w275) -> ("Error Out"=w276:errorcluster)  [unwired: 10 in, 3 out]
    }
    frame True {
    }
  }
  "error out" <- w15
